vi "UsrProfiles-Check if non-default profile.vi"() -> (3 "Non-default profile?":bool)   [LabVIEW 2017]
uses:
  Global Variables/General Globals.vi
  Globals/gl_UsrProfiles globals.vi
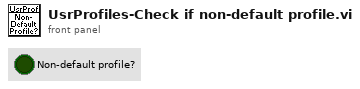
[diagram p1: front panel]
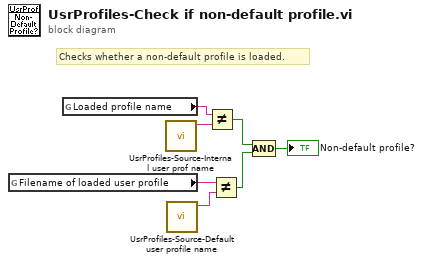
[diagram p0: block diagram]
diagram:
  # "Checks whether a non-default profile is loaded."
  n1 = global read "General Globals.vi" "Filename of loaded user profile"() -> (w1:string)
  n2 = global read "gl_UsrProfiles globals.vi" "Loaded profile name"() -> (w3:string)
  n3 = call "UsrProfiles-Source-Internal user prof name.vi"() -> ("Previous session profile name"=w4:string)  [unwired: 11 in]
  n4 = call "UsrProfiles-Source-Default user profile name.vi"() -> ("Default user's profile file name & extension"=w2:string)  [unwired: 11 in]
  n5 = Not Equal?(x=w3, y=w4) -> (x != y?=w5:bool)
  n6 = Not Equal?(x=w1, y=w2) -> (x != y?=w6:bool)
  n7 = Compound Arithmetic op=AND(w5, w6) -> (→"Non-default profile?":bool)
